vi "Tektronix_RF_scans.vi"() -> ()   [LabVIEW 2017]
panel:
  in  "VISA resource name":refnum<visa-resource-name>
  out "XY Graph 2":cluster{dbl[], dbl[]}(graph)
  out "Labels":string[](array[string])=["I_D1 (A)", "I_D2(A)", "I_SFDC (A)", "I_RF (A)", "l (mm)", "z (mm)", "Bx (mT)", "By (mT)", "Bz (mT)", "|B| (mT)"]
  in  "I_D2 (A)":dbl=112.0
  in  "I_D1 (A)":dbl=112.0
  out "Graph (Bx)":cluster{timestamp[], dbl[]}(graph)={[timestamp(3708568369.45642 s since 1904-01-01), timestamp(3708568377.924761 s since 1904-01-01)], [-0.02, -0.01]} caption="XY Graph"
  out "XY Graph":cluster{dbl[], dbl[]}(graph)
  in  "I_RF (A)":dbl=112.0
  in  "I_SFDC (A)":dbl=112.0
  out "Cycle #":i32
  in  "COMMENT":string="THM7025_zscan_practice"
  out "Graph (Bz)":cluster{timestamp[], dbl[]}(graph)={[timestamp(3708568369.45642 s since 1904-01-01), timestamp(3708568377.924761 s since 1904-01-01)], [0.25, 0.24]} caption="XY Graph"
  out "Graph (By)":cluster{timestamp[], dbl[]}(graph)={[timestamp(3708568369.45642 s since 1904-01-01), timestamp(3708568377.924761 s since 1904-01-01)], [-0.01, -0.01]} caption="XY Graph"
  in  "Stop":bool=TRUE
  out "Graph (z)":cluster{timestamp[], dbl[]}(graph)={[timestamp(3708568369.45642 s since 1904-01-01), timestamp(3708568377.924761 s since 1904-01-01)], [-0.02, -0.01]} caption="XY Graph"
  out "Z (mm) = 600 - L":dbl=378.0 format="%_5f"
  in  "L (mm)":dbl=112.0
  in  "Measure":bool
  out "File Error Out":errorcluster
  in  "base path":path=path "C:/LabVIEW/DATA/J-PARC_202206"
  in  "error in (no error)":errorcluster caption="エラー入力（エラーなし）"
  out "error out":errorcluster caption="エラー出力" {"code" format="%.0x"}
  out "Results":dbl[](array[numeric])=[-0.24, -0.01, -0.01, 0.24]
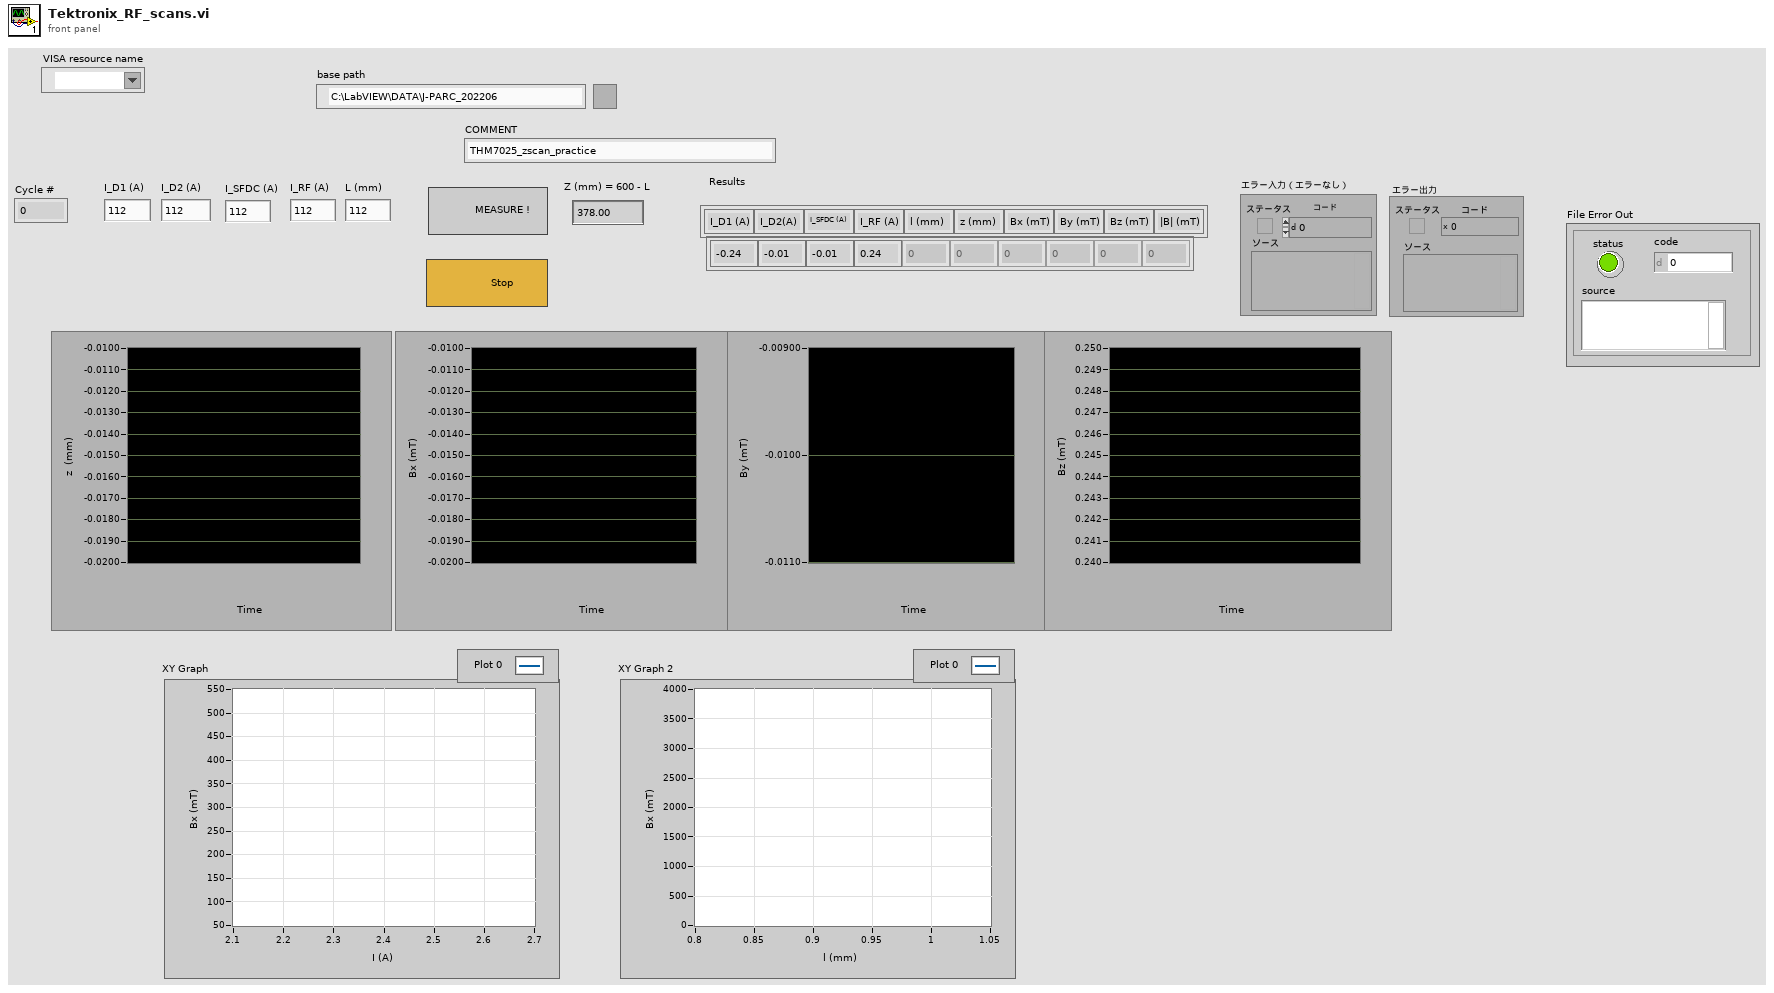
[diagram p1: front panel]
types:
  T1 = enum16{"open", "replace", "create", "open or create", "replace or create", "replace or create with confirmation"}
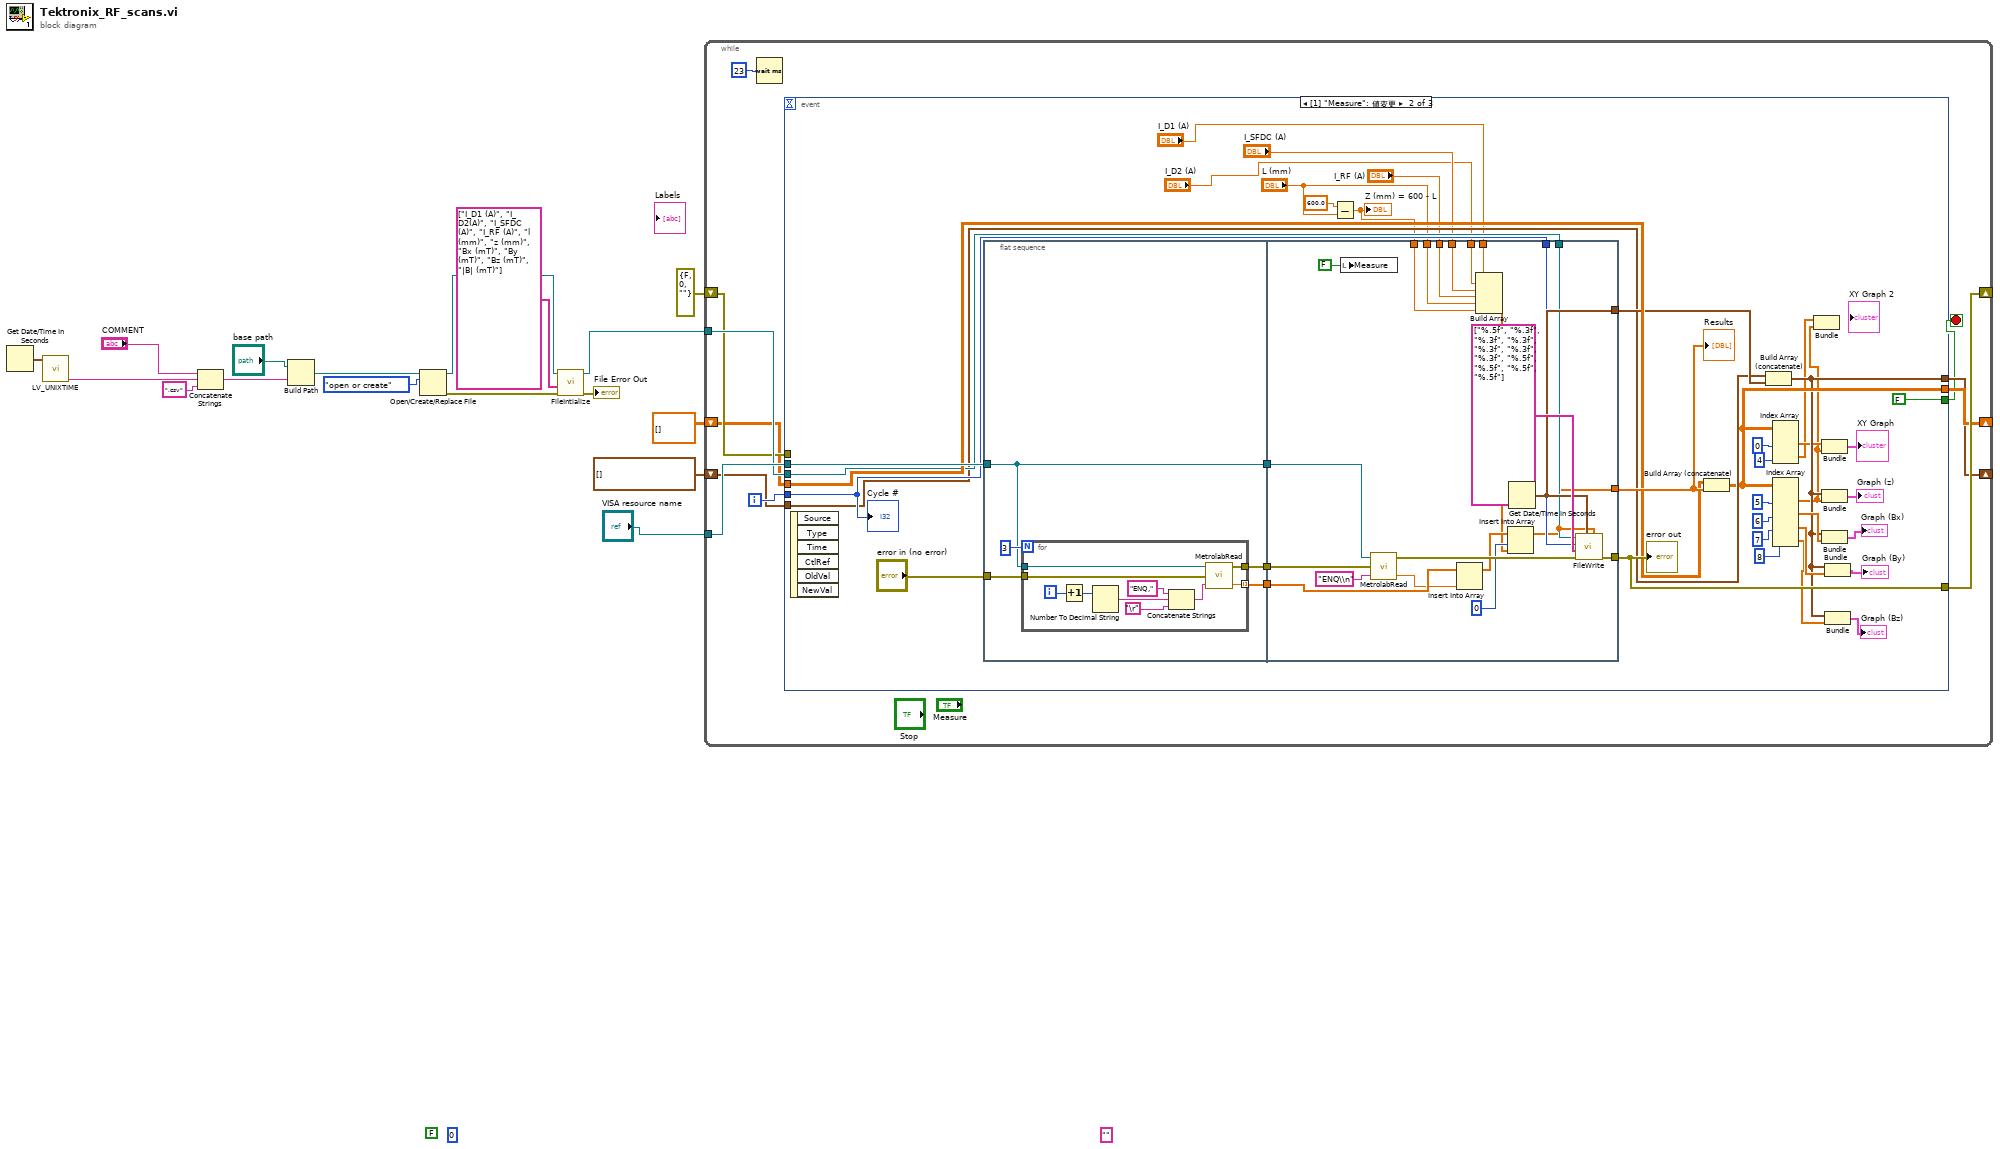
[diagram p0: block diagram]
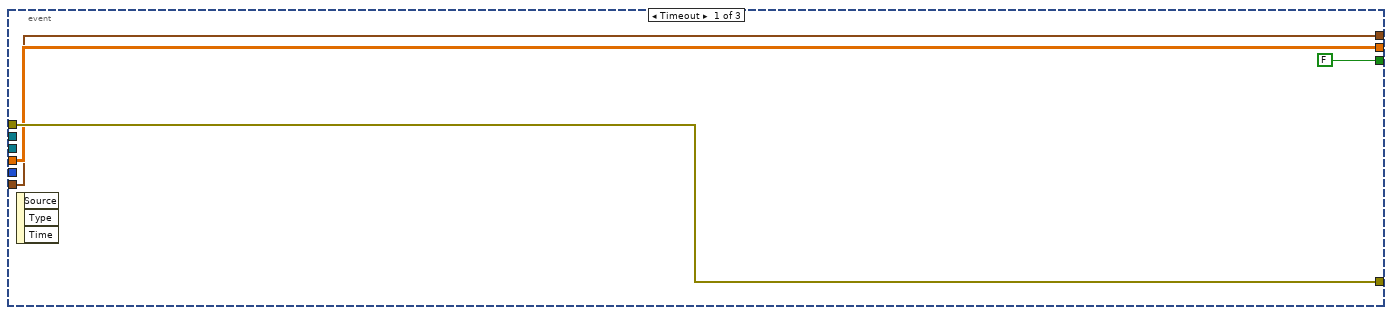
[diagram p2: hidden frame]
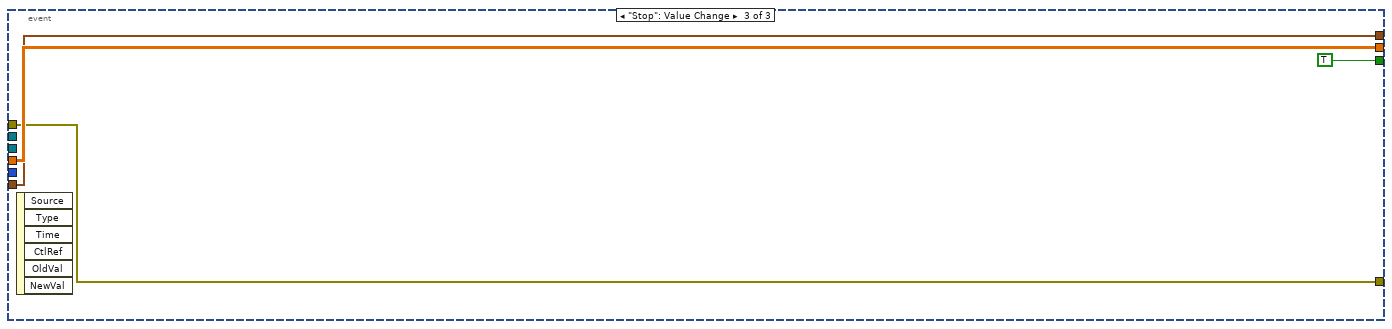
[diagram p3: hidden frame]
diagram:
  (unwired) FALSE ("status")
  (unwired) 0 ("code")
  (unwired) "" ("source")
  n1 = Get Date/Time In Seconds() -> (seconds since 1Jan1904=w15:timestamp)
  n2 = call "LV_UNIXTIME.vi"("current time"=w15) -> ("date/time string"=w12:string)  [unwired: 9 in, 1 out]
  n3 = Concatenate Strings("COMMENT", w12, ".csv" ("string")) -> (w10:string)
  n4 = Build Path(base path="base path", name or relative path=w10) -> (appended path=w14:path)
  n5 = Open/Create/Replace File(file path (use dialog)=w14, operation (0:open)=T1."open or create") -> (refnum out=w7:refnum<file>, error out=w8:errorcluster)  [unwired: 4 in, 1 out]
  n6 = call "FileIntialize.vi"("Error In"=w8, "Labels"=string[] ["I_D1 (A)", "I_D2(A)", "I_SFDC (A)", "I_RF (A)", "l (mm)", "z (mm)", "Bx (mT)", "By (mT)", "Bz (mT)", "|B| (mT)"], "refnum in"=w7) -> ("Error Out"=→"File Error Out":errorcluster, "File Refnum"=w5:refnum<file>)  [unwired: 7 in]
  n7 = while {
    tunnel: "VISA resource name" -> [w27]
    tunnel: w5 -> [w26]
    shift-right: [w24] -> _
    shift-left: errorcluster {"status"=FALSE, "code"=0, "source"=""} ("Error Out") -> [w23]
    shift-right: [w21] -> _
    shift-left: dbl[][] [] -> [w22]
    shift-right: [w20] -> _
    shift-left: timestamp[] [] -> [w19]
    i -> [w25]
    stop <- w18 stop-if-true
    n8 = Wait (ms)(milliseconds to wait=u32 23) -> ()  [unwired: 1 out]
    n9 = event shown="[1] \"Measure\": 値変更" {
      selector: _ -> [_ _ _]
      dyn-events: _ -> [_ _ _]
      timeout: _ -> [_ _ _]
      tunnel: w27 -> [_ w67 _]
      tunnel: w26 -> [_ w58 _]
      tunnel: w25 -> [_ w57 _]
      tunnel: [w32 w65 w109] -> w24
      tunnel: w23 -> [w32 _ w109]
      tunnel: w22 -> [w31 w63 w111]
      tunnel: [w31 w47 w111] -> w21
      tunnel: [w29 w39 w110] -> w20
      tunnel: w19 -> [w29 w56 w110]
      tunnel: [FALSE ("Stop") FALSE ("Stop") TRUE ("Stop")] -> w18
      event Timeout {
        n10 = event-data() -> ()  [unwired: 1 in, 3 out]
      }
      event "Measure": Value Change {
        n11 = event-data() -> ()  [unwired: 1 in, 6 out]
        n12 = flat-sequence {
          tunnel: [w72] -> w71
          tunnel: [w75] -> w70
          tunnel: [w74] -> w69
          tunnel: "error in (no error)" -> [w73]
          tunnel: w67 -> [w72]
          tunnel: w71 -> [w108]
          tunnel: w70 -> [w107]
          tunnel: w69 -> [w105]
          tunnel: [w89] -> w64
          tunnel: [w101] -> w65
          tunnel: [w100] -> w59
          tunnel: w58 -> [w99]
          tunnel: w57 -> [w98]
          tunnel: "L (mm)" -> [w97]
          tunnel: w53 -> [w96]
          tunnel: "I_SFDC (A)" -> [w92]
          tunnel: "I_RF (A)" -> [w91]
          tunnel: "I_D1 (A)" -> [w88]
          tunnel: "I_D2 (A)" -> [w87]
          frame #0 {
            n13 = for {
              N: 3 -> [_]
              tunnel: w72 -> [w86]
              tunnel: [w82] -> w74 mode=indexing
              tunnel: [w78] -> w75
              tunnel: w73 -> [w77]
              i -> [w79]
              n14 = Increment(x=w79) -> (x+1=w80:i32)
              n15 = Number To Decimal String(number=w80) -> (decimal integer string=w83:string)  [unwired: 1 in]
              n16 = Concatenate Strings("ENQ,", w83, "\r") -> (w84:string)
              n17 = call "MetrolabRead.vi"("Input string"=w84, "error in (no error)"=w77, "VISA resource name"=w86) -> ("B value [mT]"=w82:dbl, "error out"=w78:errorcluster)  [unwired: 1 out]
            }
          }
          frame #1 {
            n18 = local write "Measure"(FALSE ("Value (Signaling)")) -> ()
            n19 = call "MetrolabRead.vi"("Input string"="ENQ\\n", "error in (no error)"=w107, "VISA resource name"=w108) -> ("B value [mT]"=w104:dbl, "error out"=w102:errorcluster)  [unwired: 1 out]
            n20 = Insert Into Array(array=w105, new element=w104) -> (w93:dbl[])  [unwired: 1 in]
            n21 = Build Array(w88, w87, w92, w91, w97, w96) -> (w90:dbl[])
            n22 = Insert Into Array(array=w93, index=0, new element=w90) -> (w89:dbl[])
            n23 = Get Date/Time In Seconds() -> (seconds since 1Jan1904=w100:timestamp)
            n24 = call "FileWrite.vi"("DataArray"=w89, "Time Stamp"=w100, "Error In"=w102, "FileFormat"=string[] ["%.5f", "%.3f", "%.3f", "%.3f", "%.3f", "%.3f", "%.3f", "%.5f", "%.5f", "%.5f", "%.5f"], "Index"=w98, "refnum in"=w99) -> ("Error Out"=w101:errorcluster)  [unwired: 4 in, 1 out]
          }
        }
        n25 = Subtract(x=600.0, y="L (mm)") -> (x-y=w53:dbl)
        "Z (mm) = 600 - L" <- w53
        n26 = Build Array (concatenate)(w63, w64) -> (w47:dbl[][])
        n27 = Build Array (concatenate)(w56, w59) -> (w39:timestamp[])
        n28 = Index Array(array=w47, index (col) #1=0 ("disabled index (col)"), index (col) #2=4 ("指標 （列）")) -> (element #1=w35:dbl[], element #2=w34:dbl[])  [unwired: 2 in]
        n29 = Index Array(array=w47, index (col) #1=5 ("disabled index (col)"), index (col) #2=6 ("disabled index (col)"), index (col) #3=7 ("disabled index (col)"), index (col) #4=8 ("index (col)")) -> (element #1=w33:dbl[], element #2=w51:dbl[], element #3=w50:dbl[], element #4=w43:dbl[])  [unwired: 4 in]
        n30 = Bundle(w34, w33) -> ()  [unwired: 1 in, 1 out]
        n31 = Bundle(w35, w33) -> (→"XY Graph":cluster{dbl[], dbl[]})  [unwired: 1 in]
        n32 = Bundle(w39, w33) -> (→"Graph (z)":cluster{timestamp[], dbl[]})  [unwired: 1 in]
        n33 = Bundle(w39, w51) -> (→"Graph (Bx)":cluster{timestamp[], dbl[]})  [unwired: 1 in]
        n34 = Bundle(w39, w50) -> (→"Graph (By)":cluster{timestamp[], dbl[]})  [unwired: 1 in]
        n35 = Bundle(w39, w43) -> (→"Graph (Bz)":cluster{timestamp[], dbl[]})  [unwired: 1 in]
        "Results" <- w64
        "error out" <- w65
        "Cycle #" <- w57
      }
      event "Stop": Value Change {
        n36 = event-data() -> ()  [unwired: 1 in, 6 out]
      }
    }
  }
